vi "Launcher - UserInterface.vi"() -> ()   [LabVIEW 2021]
uses:
  Workers/UserInterface/UserInterface.lvclass
  C:/Program Files (x86)/National Instruments/LabVIEW 2021/vi.lib/addons/_Workers/Library/Classes/Worker/Worker.lvclass
  <vilib>/addons/_Workers/Debugger/Debug Client/Debug Client.lvlib
panel:
  out "error out":errorcluster
  in  "error in":errorcluster
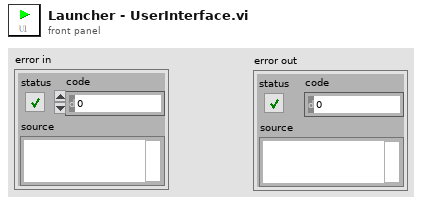
[diagram p1: front panel]
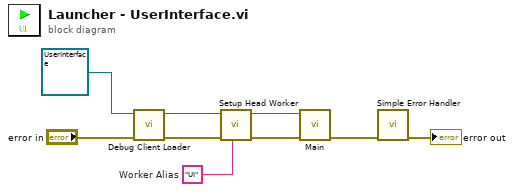
[diagram p0: block diagram]
diagram:
  w4 = "UI"  # Worker Alias
  n1 = call <vilib>:"Debug Client Loader.vi"("error in (no error)"="error in", "Worker"=refnum<class "UserInterface.lvclass"> refnum ("Worker User Object")) -> ("error out"=w3:errorcluster, "Worker out"=w1:refnum<class "UserInterface.lvclass">)  [unwired: 8 in]
  n2 = call-dynamic "Setup Head Worker.vi"("Worker Alias"=w4, "error in"=w3, "Worker"=w1) -> ("error out"=w9:errorcluster, "Worker out"=w6:refnum<class "UserInterface.lvclass">)  [unwired: 7 in]
  n3 = call-dynamic "Main.vi"("error in"=w9, "UserInterface in"=w6) -> ("error out"=w7:errorcluster)  [unwired: 8 in, 1 out]
  n4 = call <vilib>:"Simple Error Handler.vi"("error in (no error)"=w7) -> ("error out"=→"error out":errorcluster)  [unwired: 4 in, 4 out]
